vi "SRS Select Model.vi"(10 "Model":string, 11 "Instruments in":T1[](array[typedef])) -> (3 "Instruments out":T1[](array[typedef]))   [LabVIEW 2024]
uses:
  Sub Controls/Instrument Match.ctl
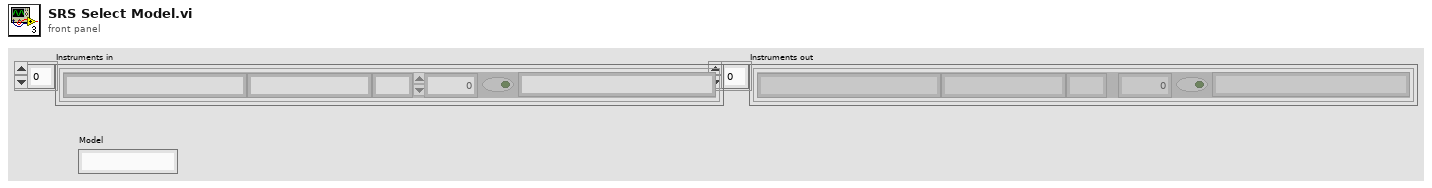
[diagram p1: front panel]
types:
  T1 = typedef "Instrument Match.ctl" = cluster{"Model":string, "Manufacturer":string, "Term Character":string, "Wait Time (mS)":u32, "Wait for SRQ":bool, "Type":string}
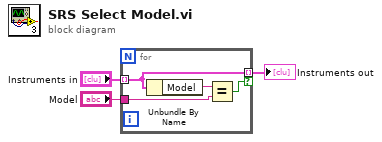
[diagram p0: block diagram]
diagram:
  n1 = for {
    tunnel: "Instruments in" -> [w7] mode=indexing
    tunnel: [w7] -> w2 mode=indexing if=w4
    tunnel: "Model" -> [w6]
    n2 = Unbundle By Name(w7) -> ("Model"=w5:string)
    n3 = Equal?(x=w5, y=w6) -> (x = y?=w4:bool)
  }
  "Instruments out" <- w2
